vi "Halfwave Model.vi"(6 "Ignore Offset":bool, 8 "Length":i32, 9 "Sample Rate":i32, 10 "Phase (deg)":dbl, 11 "Frequency":dbl) -> (3 "Array":dbl[][](array[numeric]))   [LabVIEW 2016, in "Halfwave Sinusoidal Fit.lvclass"]
uses:
  Halfwave Sinusoidal Fit.lvclass
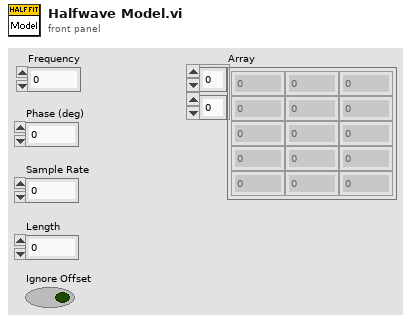
[diagram p1: front panel]
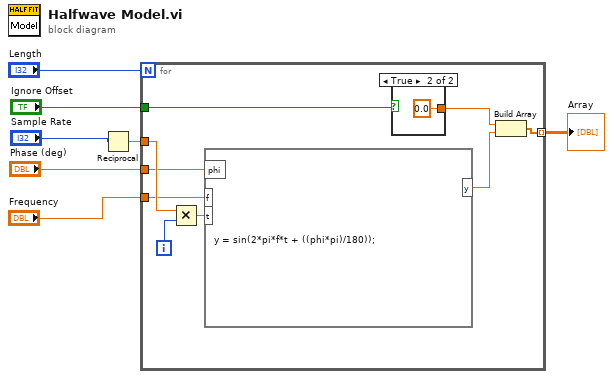
[diagram p0: block diagram]
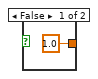
[diagram p2: hidden frame]
diagram:
  n1 = Reciprocal(x="Sample Rate") -> (1/x=w4:dbl)
  n2 = for {
    N: "Length" -> [_]
    tunnel: [w15] -> w6 mode=indexing
    tunnel: w4 -> [w14]
    tunnel: "Frequency" -> [w12]
    tunnel: "Phase (deg)" -> [w10]
    tunnel: "Ignore Offset" -> [w8]
    i -> [w16]
    n3 = Multiply(x=w14, y=w16) -> (x*y=w13:dbl)
    n4 = formula code="y = sin(2*pi*f*t + ((phi*pi)/180));"("t"=w13, "f"=w12, "phi"=w10) -> ("y"=w11:dbl)
    n5 = case shown="True" w8 {
      tunnel: [1.0 ("element") 0.0 ("element")] -> w9
      frame False {
      }
      frame True {
      }
    }
    n6 = Build Array(w9, w11) -> (w15:dbl[])
  }
  "Array" <- w6
